vi "ModbusCRC16.vi"(4 "Data":string) -> (1 "CRC16":string)   [LabVIEW 2020]
doc: "RTU 检查码(CRC)计算, 运算规则如下:\n步骤1: 令16-bit 暂存器(CRC 暂存器) = 0xFFFF。\n步骤2: Exclusive OR 第一个8-bit byte 的讯息指令与低位元16-bit CRC 暂存器, 做Exclusive OR 将结果存入CRC 暂存器内。\n步骤3: 右移一位CRC 暂存器, 将0 填入高位元处。\n步骤4: 检查右移的值, 如果是0 将步骤3 的新值存入CRC 暂存器内, 否则Exclusive OR 0xA001 与CRC 暂存器, 将结果存入CRC 暂存器内。\n步骤5: 重复步骤3~步骤4, 将8-bit 全部运算完成。\n步骤6: 重复步骤2~步骤5, 取下一个8-bit 的讯息指令, 直到所有讯息指令运算完成。最后, 得到的CRC 暂存器的值, 即是CRC 的检查码。值得注意的是CRC 的检查码必须交换放置于讯息指令的检查码中。"
panel:
  # "RTU 检查码(CRC)计算, 运算规则如下:\n步骤1: 令16-bit 暂存器(CRC 暂存器) = 0xFFFF。\n步骤2: Exclusive OR 第一个8-bit byte 的讯息指令与低位元16-bit CRC 暂存器, 做Exclusive OR 将结果存入CRC 暂存器内。\n步骤3: 右移一位CRC 暂存器, 将0 填入高位元处。\n步骤4: 检查右移的值, 如果是0 将步骤3 的新值存入CRC 暂存器内, 否则Exclusive OR 0xA001 与CRC 暂存器, 将结果存入CRC 暂存器内。\n步骤5: 重复步骤3~步骤4, 将8-bit 全部运算完成。\n步骤6: 重复步骤2~步骤5, 取下一个8-bit 的讯息指令, 直到所有讯息指令运算完成。最后, 得到的CRC 暂存器的值, 即是CRC 的检查码。值得注意的是CRC 的检查码必须交换放置于讯息指令的检查码中。"
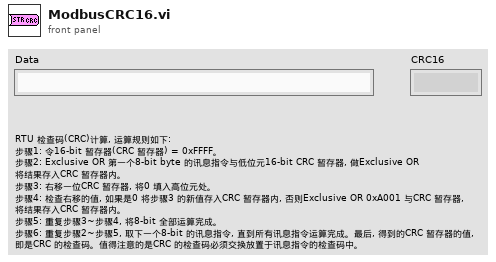
[diagram p1: front panel]
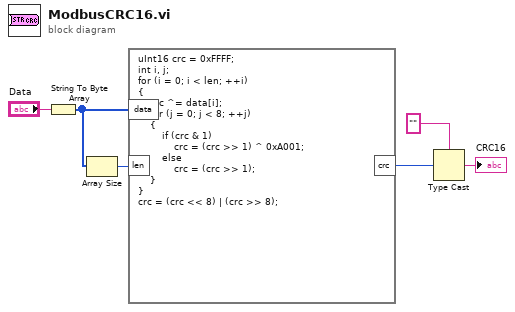
[diagram p0: block diagram]
diagram:
  n1 = String To Byte Array(string="Data") -> (unsigned byte array=w5:u8[])
  n2 = Array Size(array=w5) -> (size(s)=w4:i32)
  n3 = formula code="uInt16 crc = 0xFFFF;\nint i, j;\nfor (i = 0; i < len; ++i)\n{\n    crc ^= data[i];\n    for (j = 0; j < 8; ++j)\n    {\n        if (crc & 1)\n            crc = (crc >> 1) ^ 0xA001;\n        else\n            crc = (crc >> 1);\n    }\n}\ncrc = (crc << 8) | (crc >> 8);"("data"=w5, "len"=w4) -> ("crc"=w1:u16)
  n4 = Type Cast(type="" ("类型"), x=w1) -> (*(type *) &x=→"CRC16":string)
